vi "AD9910 Register Info.vi"(10 "Register":T1) -> (1 "Number of Bytes":i32, 2 "Address":u8)   [LabVIEW 2013]
doc: "Returns the address and number of bytes in a given AD9910 register."
uses:
  AD9910 registers.ctl
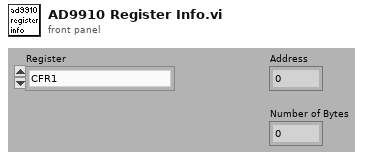
[diagram p1: front panel]
types:
  T1 = typedef "AD9910 registers.ctl" = enum16{"CFR1", "CFR2", "CFR3", "Auxiliary DAC Control", "I/0 Update Rate", "Frequency Tuning Word", "Phase Offset Word", "Amplitude Scale Factor", "Multichip Sync", "Digital Ramp Limit", "Digital Ramp Step Size", "Digital Ramp Rate", "Single Tone Profile 0", "Single Tone Profile 1", "Single Tone Profile 2", "Single Tone Profile 3", "Single Tone Profile 4", "Single Tone Profile 5", "Single Tone Profile 6", "Single Tone Profile 7", "RAM Profile 0", "RAM Profile 1", "RAM Profile 2", "RAM Profile 3", "RAM Profile 4", "RAM Profile 5", "RAM Profile 6", "RAM Profile 7", "RAM"}
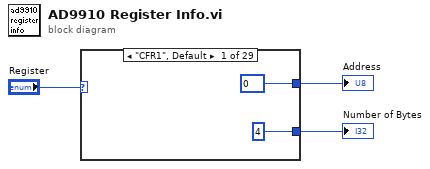
[diagram p0: block diagram]
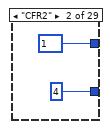
[diagram p2: hidden frame]
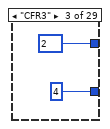
[diagram p3: hidden frame]
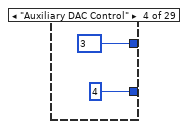
[diagram p4: hidden frame]
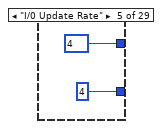
[diagram p5: hidden frame]
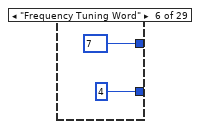
[diagram p6: hidden frame]
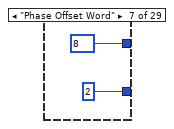
[diagram p7: hidden frame]
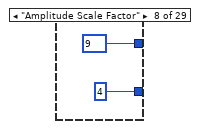
[diagram p8: hidden frame]
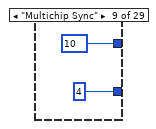
[diagram p9: hidden frame]
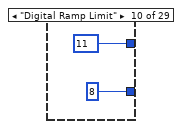
[diagram p10: hidden frame]
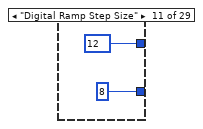
[diagram p11: hidden frame]
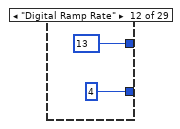
[diagram p12: hidden frame]
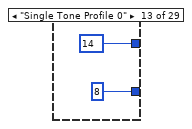
[diagram p13: hidden frame]
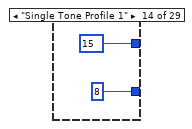
[diagram p14: hidden frame]
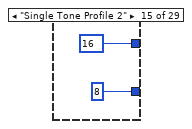
[diagram p15: hidden frame]
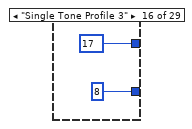
[diagram p16: hidden frame]
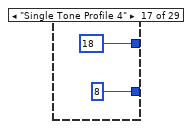
[diagram p17: hidden frame]
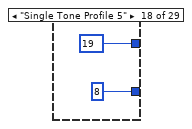
[diagram p18: hidden frame]
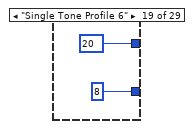
[diagram p19: hidden frame]
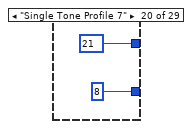
[diagram p20: hidden frame]
diagram:
  n1 = case shown="\"CFR1\", Default" "Register" {
    tunnel: [u8 0 u8 1 u8 2 u8 3 u8 4 u8 7 u8 8 u8 9 u8 10 u8 11 u8 12 u8 13 u8 14 u8 15 u8 16 u8 17 u8 18 u8 19 u8 20 u8 21 u8 14 u8 15 u8 16 u8 17 u8 18 u8 19 u8 20 u8 21 u8 22] -> w2
    tunnel: [u8 4 u8 4 u8 4 u8 4 u8 4 u8 4 u8 2 u8 4 u8 4 u8 8 u8 8 u8 4 u8 8 u8 8 u8 8 u8 8 u8 8 u8 8 u8 8 u8 8 u8 8 u8 8 u8 8 u8 8 u8 8 u8 8 u8 8 u8 8 u8 4] -> w1
    frame "CFR1", Default {
    }
    frame "CFR2" {
    }
    frame "CFR3" {
    }
    frame "Auxiliary DAC Control" {
    }
    frame "I/0 Update Rate" {
    }
    frame "Frequency Tuning Word" {
    }
    frame "Phase Offset Word" {
    }
    frame "Amplitude Scale Factor" {
    }
    frame "Multichip Sync" {
    }
    frame "Digital Ramp Limit" {
    }
    frame "Digital Ramp Step Size" {
    }
    frame "Digital Ramp Rate" {
    }
    frame "Single Tone Profile 0" {
    }
    frame "Single Tone Profile 1" {
    }
    frame "Single Tone Profile 2" {
    }
    frame "Single Tone Profile 3" {
    }
    frame "Single Tone Profile 4" {
    }
    frame "Single Tone Profile 5" {
    }
    frame "Single Tone Profile 6" {
    }
    frame "Single Tone Profile 7" {
    }
    frame "RAM Profile 0" {
    }
    frame "RAM Profile 1" {
    }
    frame "RAM Profile 2" {
    }
    frame "RAM Profile 3" {
    }
    frame "RAM Profile 4" {
    }
    frame "RAM Profile 5" {
    }
    frame "RAM Profile 6" {
    }
    frame "RAM Profile 7" {
    }
    frame "RAM" {
    }
  }
  "Address" <- w2
  "Number of Bytes" <- w1
